vi "NISE.remote.Initialize (Core).vi"(0 "resources":string, 1 "Hostname/IP":string, 2 "Port":u16, 3 "https?":bool, 5 "slsc type":T1, 7 "reservation access (Read/Write)":i32(ring)=3 items=["None"=0, "Read Only"=1, "Read/Write"=3], 9 "reservation group":string, 11 "error in (no error)":errorcluster, 12 "connect timeout (60 sec)":dbl=60.0, 13 "username":string, 14 "password":string) -> (4 "SLSC Remote out":refnum<class "SLSC Interface.lvclass">, 15 "error out":errorcluster)   [LabVIEW 2016, in "SLSC Interface.lvclass"]
uses:
  SLSC Interface Class/SLSC Interface.lvclass
  SLSC Interface Class/NISE.slsc type.ctl
  SLSC Interface Class/SLSC Interface.lvclass/SLSC Interface.ctl
  SLSC Interface Class/NISE.Write URL.vi
  SLSC Interface Class/NISE.Write client handle.vi
  <vilib>/httpClient/POSTBuffer.vi
  <vilib>/NI/JSON Support for LabVIEW/JSON Value/Object/Get Value/Get Value (String).vi
  SLSC Interface Class/NISE.Write session.vi
  <vilib>/httpClient/LabVIEWHTTPClient.lvlib
  <vilib>/NI/JSON Support for LabVIEW/JSON Value/JSON Value.lvclass
  <vilib>/NI/NI JSONRPC Server Framework/Classes/Client/JSONRPC Client.lvclass
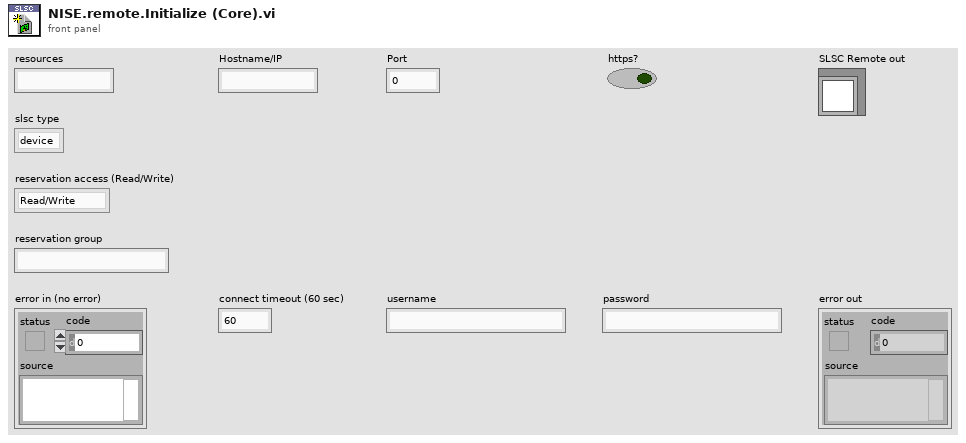
[diagram p1: front panel]
types:
  T1 = typedef "SLSC Interface.lvclass/NISE.slsc type.ctl" = enum16{"device", "nvmem", "channel", "none"}
  T2 = typedef "LabVIEWHTTPClient.lvlib/ClientHandle.ctl" = refnum<k1>
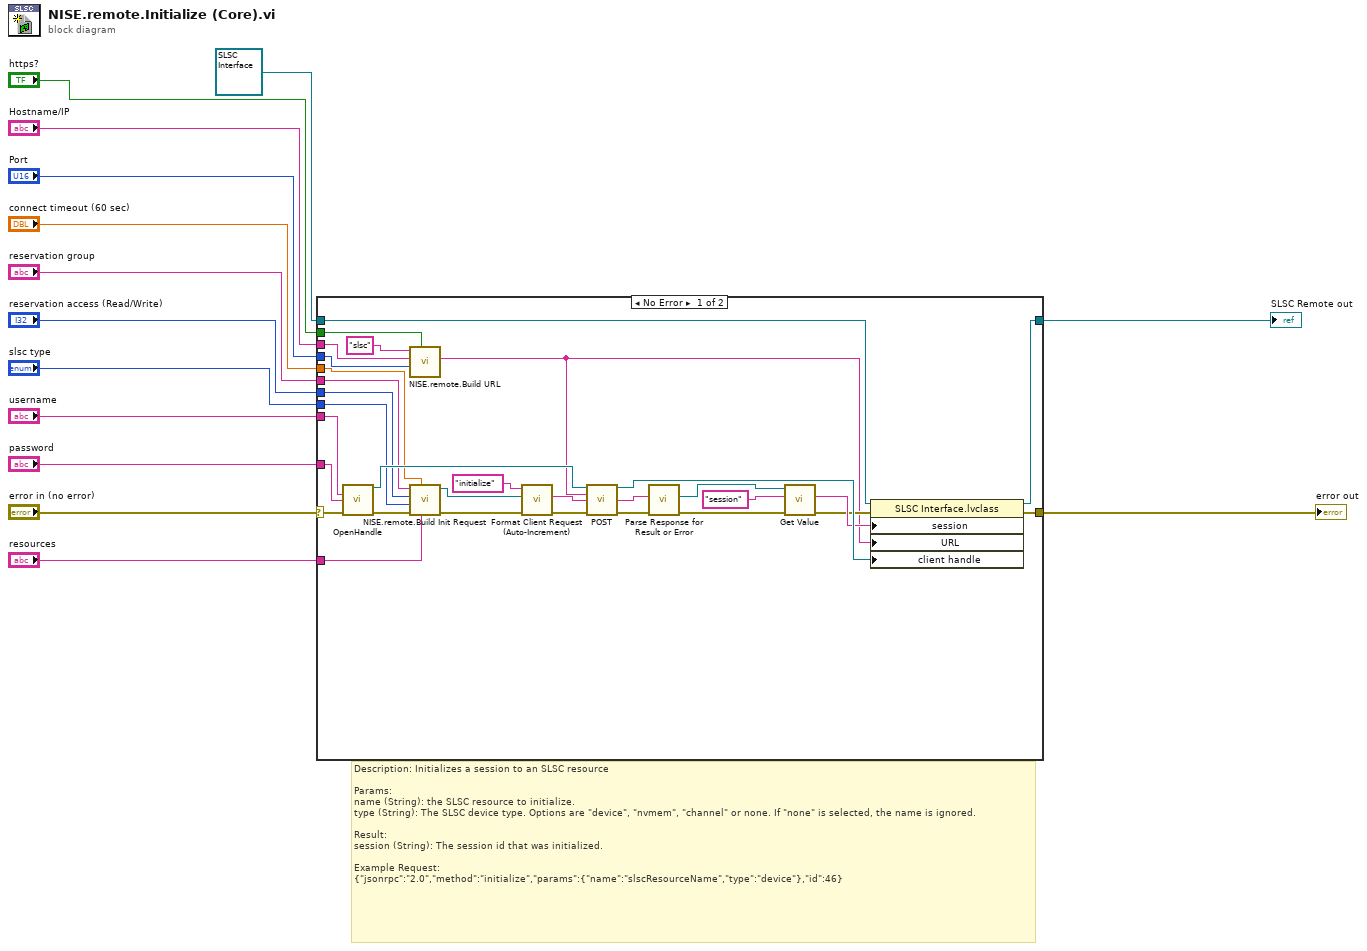
[diagram p0: block diagram]
diagram:
  # "Description: Initializes a session to an SLSC resource\n\nParams:\nname (String): the SLSC resource to initialize.\ntype (String): The SLSC device type. Options are \"device\", \"nvmem\", \"channel\" or none. If \"none\" is selected, the name is ignored.\n\nResult:\nsession (String): The session id that was initialized.\n\nExample Request: \n{\"jsonrpc\":\"2.0\",\"method\":\"initialize\",\"params\":{\"name\":\"slscResourceName\",\"type\":\"device\"},\"id\":46}"
  n1 = case shown="No Error" "error in (no error)" {
    selector: "error in (no error)" -> [w40 w47]
    tunnel: [w43 w47] -> w14
    tunnel: [w44 w46] -> w13
    tunnel: refnum<class "SLSC Interface.lvclass"> refnum ("SLSC Interfaces.lvlib:SLSC Interface.lvclass") -> [w45 w46]
    tunnel: "resources" -> [w23 _]
    tunnel: "username" -> [w42 _]
    tunnel: "password" -> [w41 _]
    tunnel: "https?" -> [w35 _]
    tunnel: "Hostname/IP" -> [w34 _]
    tunnel: "Port" -> [w33 _]
    tunnel: "slsc type" -> [w24 _]
    tunnel: "reservation access (Read/Write)" -> [w21 _]
    tunnel: "reservation group" -> [w20 _]
    tunnel: "connect timeout (60 sec)" -> [w19 _]
    frame No Error {
      n2 = call <vilib>:"OpenHandle.vi"("username"=w42, "password"=w41, "error in (no error)"=w40) -> ("client handle out"=w39:T2, "error out"=w22:errorcluster)  [unwired: 11 in]
      n3 = call "NISE.remote.Build URL.vi"("https?"=w35, "Port"=w33, "Hostname/IP"=w34, "service name"="slsc") -> ("URL"=w32:string)  [unwired: 7 in]
      n4 = call "NISE.remote.Build Init Request.vi"("resource"=w23, "connect timeout"=w19, "error in (no error)"=w22, "slsc type"=w24, "reservation access"=w21, "reservation group"=w20) -> ("error out"=w17:errorcluster, "JSON Value out"=w18:refnum<class "JSON Value.lvclass">)  [unwired: 4 in]
      n5 = call <vilib>:"Format Client Request (Auto-Increment).vi"("error in (no error)"=w17, "JSON Value in"=w18, "method"="initialize") -> ("error out"=w16:errorcluster, "Request String"=w25:string)  [unwired: 7 in]
      n6 = call-poly <vilib>:"POST.vi"("client handle"=w39, "url"=w32, "buffer"=w25, "error in (no error)"=w16) -> ("client handle out"=w38:T2, "body"=w31:string, "error out"=w28:errorcluster)  [unwired: 8 in, 1 out]
      n7 = call <vilib>:"Parse Response for Result or Error.vi"("error in"=w28, "Response String In"=w31) -> ("error out"=w29:errorcluster, "JSON Value out"=w15:refnum<class "JSON Value.lvclass">)  [unwired: 7 in, 1 out]
      n8 = call-poly <vilib>:"Get Value.vi"("error in (no error)"=w29, "key"="session" ("Parameter Name"), "JSON Value in"=w15) -> ("error out"=w36:errorcluster, "value"=w37:string)  [unwired: 7 in]
      n9 = property class="SLSC Interface.lvclass"(reference=w45, error in=w36, "session"=w37, "URL"=w32, "client handle"=w38) -> (reference out=w44:refnum<class "SLSC Interface.lvclass">, error out=w43:errorcluster)
    }
    frame Error {
    }
  }
  "error out" <- w14
  "SLSC Remote out" <- w13
